vi "Untitled 1.vi"() -> ()   [LabVIEW 2020]
uses:
  <vilib>/Instr/_visa.llb/VISA Configure Serial Port (Instr).vi
panel:
  out "z":string
  out "y":string
  out "x":string
  out "y":i32(graph)
  out "x":i32(graph)
  out "z":i32=61
  out "y":i32=61
  out "z":i32(graph)
  in  "等待时间(ms)":u32=200
  out "缓存区":string="23161"
  in  "字节数(5)":u32=5
  in  "开关":bool=TRUE
  out "x":i32=61
  out "错误输出":cluster{"status":bool, i32, string}={"status"=FALSE, 1073676294, "VISA Read in Untitled 1.vi"}
  in  "串口":refnum<visa-resource-name>="COM4"
  in  "串口设置":T1={"流控制 (0:none)"=0, "停止位 (10: 1 bit)"=10, "奇偶校验 (0:none)"=0, "数据比特 (8)"=8, "比特率 (115200)"=115200} {"数据比特 (8)" min=5 max=8 step=1; "奇偶校验 (0:none)" items=["None", "Odd", "Even", "Mark", "Space"]; "流控制 (0:none)" items=["None", "XON/XOFF", "RTS/CTS", "XON/XOFF & RTS/CTS", "DTR/DSR", "XON/XOFF & DTR/DSR"]}
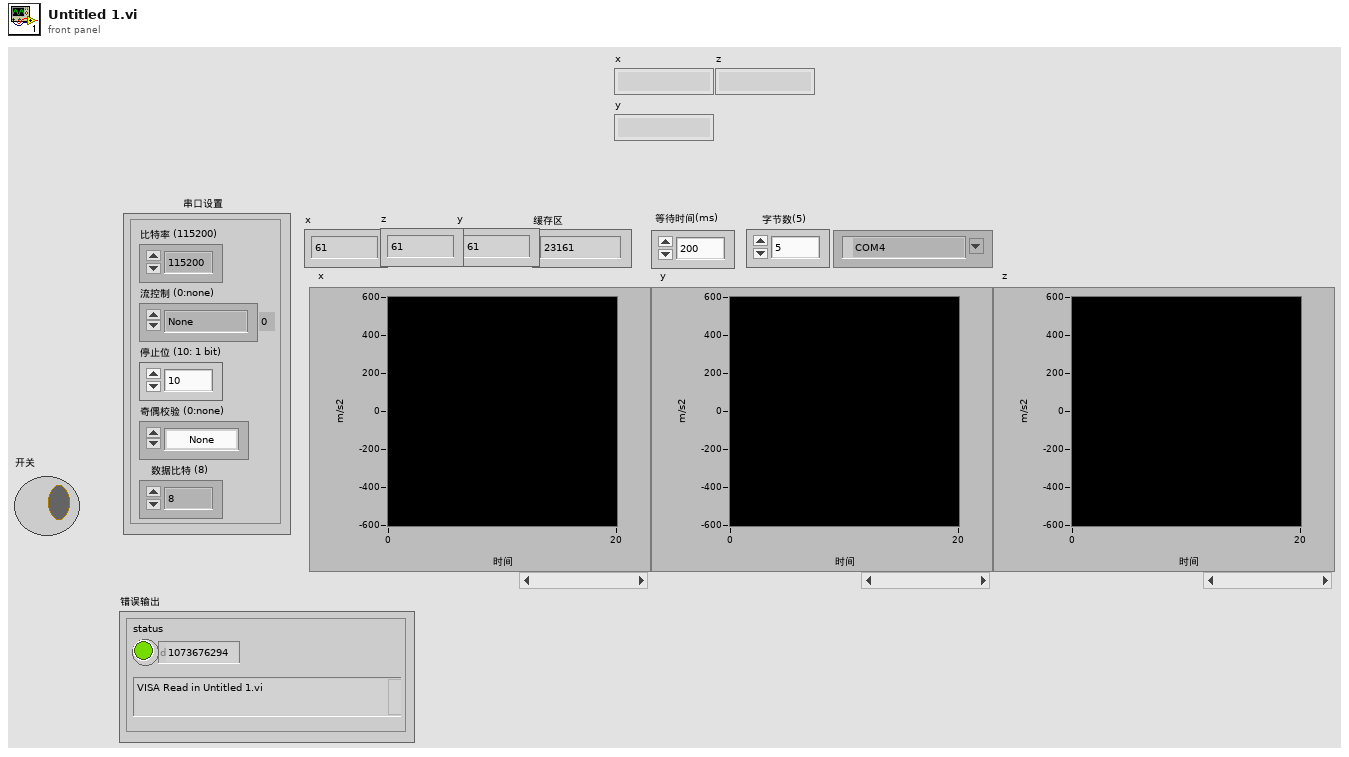
[diagram p1: front panel]
types:
  T1 = cluster{"流控制 (0:none)":u16, "停止位 (10: 1 bit)":u16, "奇偶校验 (0:none)":u16, "数据比特 (8)":u16, "比特率 (115200)":u32}
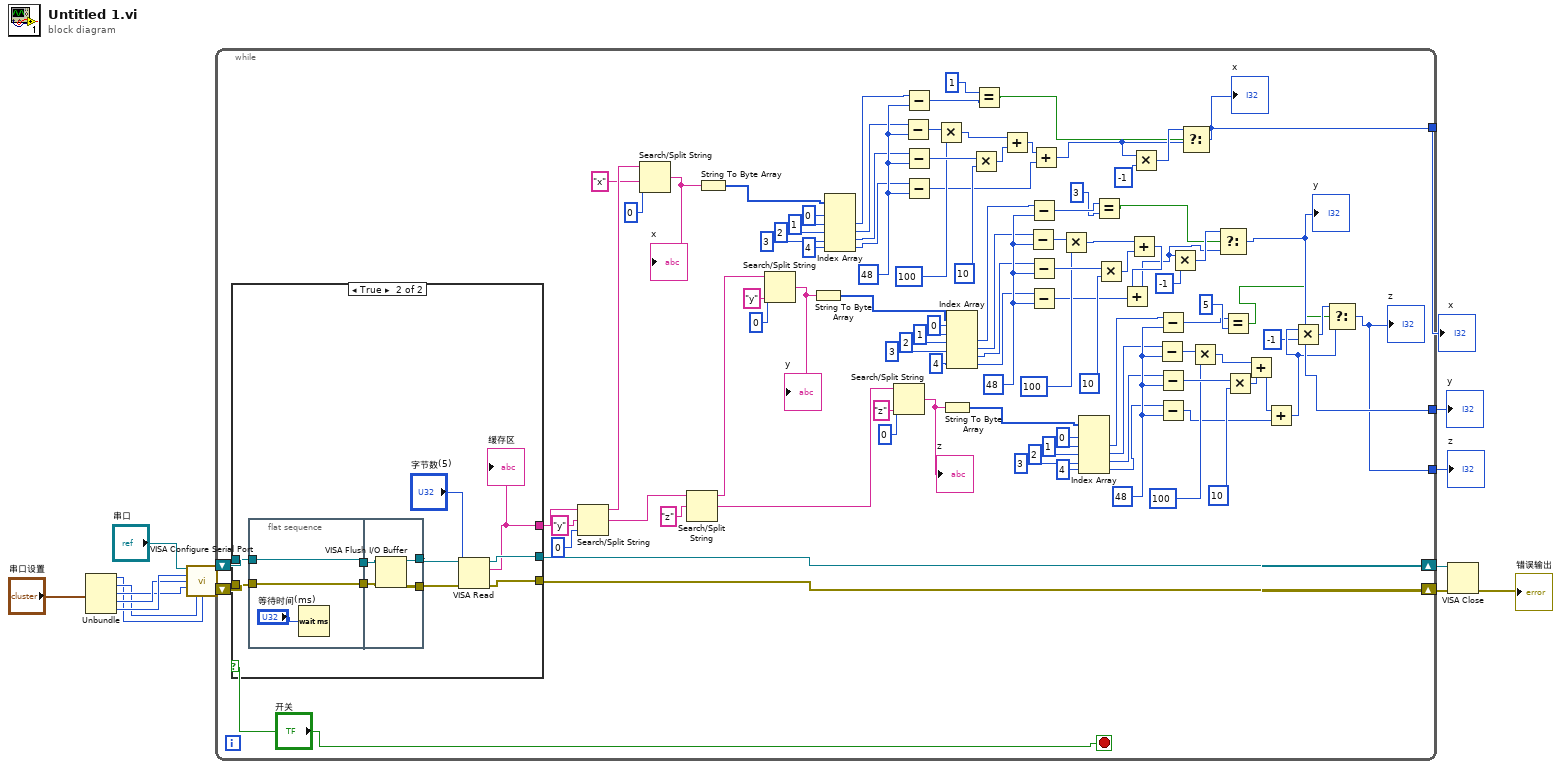
[diagram p0: block diagram]
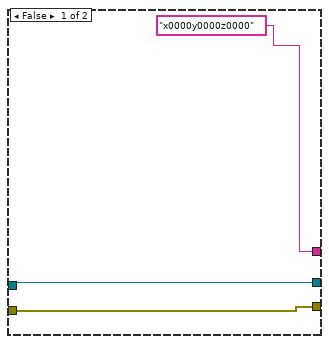
[diagram p2: hidden frame]
diagram:
  n1 = Unbundle("串口设置") -> ("流控制 (0:none)"=w7:u16, "停止位 (10: 1 bit)"=w8:u16, "奇偶校验 (0:none)"=w9:u16, "数据比特 (8)"=w10:u16, "比特率 (115200)"=w11:u32)
  n2 = call-poly "VISA Configure Serial Port"("VISA resource name"="串口", "baud rate (9600)"=w11, "data bits (8)"=w10, "parity (0:none)"=w9, "stop bits (10: 1 bit)"=w8, "flow control (0:none)"=w7) -> ("VISA resource name out"=w15:refnum<visa-resource-name>, "error out"=w14:errorcluster)  [unwired: 8 in]
  n3 = while {
    shift-right: [w112] -> w5
    shift-left: w15 -> [w115]
    shift-right: [w113] -> w6
    shift-left: w14 -> [w114]
    tunnel: [w53] -> w3
    tunnel: [w52] -> w2
    tunnel: [w51] -> w1
    stop <- "开关" stop-if-true
    w72 = 48
    w87 = 48
    w105 = 48
    n4 = case shown="True" "开关" {
      tunnel: w115 -> [w118 w126]
      tunnel: w114 -> [w117 w125]
      tunnel: [w117 w124] -> w113
      tunnel: [w118 w123] -> w112
      tunnel: ["x0000y0000z0000" ("read buffer") w119] -> w98
      frame False {
      }
      frame True {
        n5 = flat-sequence {
          tunnel: [w131] -> w128
          tunnel: w126 -> [w131]
          tunnel: w125 -> [w130]
          tunnel: [w130] -> w127
          tunnel: [w135] -> w121
          tunnel: w128 -> [w134]
          tunnel: w127 -> [w133]
          tunnel: [w132] -> w122
          frame #0 {
            n6 = Wait (ms)(milliseconds to wait="等待时间(ms)") -> ()  [unwired: 1 out]
          }
          frame #1 {
            n7 = VISA Flush I/O Buffer(VISA resource name=w134, error in (no error)=w133) -> (VISA resource name out=w135:refnum<visa-resource-name>, error out=w132:errorcluster)  [unwired: 1 in]
          }
        }
        n8 = VISA Read(VISA resource name=w121, byte count="字节数(5)", error in (no error)=w122) -> (VISA resource name out=w123:refnum<visa-resource-name>, read buffer=w119:string, error out=w124:errorcluster)  [unwired: 1 out]
        "缓存区" <- w119
      }
    }
    n9 = Search/Split String(string=w98, search string/char (-)="y", offset (0)=0) -> (substring before match=w95:string, match + rest of string=w62:string)  [unwired: 1 out]
    n10 = Search/Split String(string=w95, search string/char (-)="x", offset (0)=0) -> (match + rest of string=w40:string)  [unwired: 2 out]
    "x" <- w40
    n11 = Search/Split String(string=w62, search string/char (-)="z") -> (substring before match=w60:string, match + rest of string=w59:string)  [unwired: 1 in, 1 out]
    n12 = String To Byte Array(string=w40) -> (unsigned byte array=w106:u8[])
    n13 = Search/Split String(string=w60, search string/char (-)="y", offset (0)=0) -> (match + rest of string=w78:string)  [unwired: 2 out]
    "y" <- w78
    n14 = String To Byte Array(string=w78) -> (unsigned byte array=w88:u8[])
    n15 = Index Array(array=w106, index #1=0 ("index"), index #2=1 ("index"), index #3=2 ("index"), index #4=3 ("index"), index #5=4 ("index")) -> (element #2=w36:u8, element #3=w35:u8, element #4=w33:u8, element #5=w34:u8)  [unwired: 1 out]
    n16 = Search/Split String(string=w59, search string/char (-)="z", offset (0)=0) -> (match + rest of string=w63:string)  [unwired: 2 out]
    "z" <- w63
    n17 = Subtract(x=w35, y=w105) -> (x-y=w104:i32)
    n18 = Subtract(x=w36, y=w105) -> (x-y=w23:i32)
    n19 = Subtract(x=w33, y=w105) -> (x-y=w103:i32)
    n20 = Subtract(x=w34, y=w105) -> (x-y=w50:i32)
    n21 = Multiply(x=w104, y=100) -> (x*y=w100:i32)
    n22 = String To Byte Array(string=w63) -> (unsigned byte array=w73:u8[])
    n23 = Index Array(array=w88, index #1=0 ("index"), index #2=1 ("index"), index #3=2 ("index"), index #4=3 ("index"), index #5=4 ("index")) -> (element #2=w32:u8, element #3=w31:u8, element #4=w30:u8, element #5=w29:u8)  [unwired: 1 out]
    n24 = Multiply(x=w103, y=10) -> (x*y=w99:i32)
    n25 = Equal?(x=1 ("y"), y=w23) -> (x = y?=w22:bool)
    n26 = Add(x=w100, y=w99) -> (x+y=w49:i32)
    n27 = Subtract(x=w31, y=w87) -> (x-y=w86:i32)
    n28 = Subtract(x=w32, y=w87) -> (x-y=w21:i32)
    n29 = Subtract(x=w30, y=w87) -> (x-y=w85:i32)
    n30 = Subtract(x=w29, y=w87) -> (x-y=w47:i32)
    n31 = Add(x=w49, y=w50) -> (x+y=w48:i32)
    n32 = Multiply(x=w86, y=100) -> (x*y=w82:i32)
    n33 = Index Array(array=w73, index #1=0 ("index"), index #2=1 ("index"), index #3=2 ("index"), index #4=3 ("index"), index #5=4 ("index")) -> (element #2=w28:u8, element #3=w27:u8, element #4=w26:u8, element #5=w25:u8)  [unwired: 1 out]
    n34 = Equal?(x=w21, y=3) -> (x = y?=w19:bool)
    n35 = Multiply(x=w85, y=10) -> (x*y=w81:i32)
    n36 = Add(x=w82, y=w81) -> (x+y=w46:i32)
    n37 = Add(x=w46, y=w47) -> (x+y=w45:i32)
    n38 = Multiply(x=w48, y=-1) -> (x*y=w57:i32)
    n39 = Subtract(x=w27, y=w72) -> (x-y=w71:i32)
    n40 = Subtract(x=w28, y=w72) -> (x-y=w16:i32)
    n41 = Subtract(x=w26, y=w72) -> (x-y=w70:i32)
    n42 = Subtract(x=w25, y=w72) -> (x-y=w44:i32)
    n43 = Multiply(x=w45, y=-1) -> (x*y=w56:i32)
    n44 = Select(t=w57, s=w22, f=w48) -> (s? t:f=w53:i32)
    "x" <- w53
    n45 = Multiply(x=w71, y=100) -> (x*y=w67:i32)
    n46 = Select(t=w56, s=w19, f=w45) -> (s? t:f=w52:i32)
    "y" <- w52
    n47 = Equal?(x=w16, y=5) -> (x = y?=w18:bool)
    n48 = Multiply(x=w70, y=10) -> (x*y=w66:i32)
    n49 = Add(x=w67, y=w66) -> (x+y=w43:i32)
    n50 = Add(x=w43, y=w44) -> (x+y=w42:i32)
    n51 = Multiply(x=w42, y=-1) -> (x*y=w54:i32)
    n52 = Select(t=w54, s=w18, f=w42) -> (s? t:f=w51:i32)
    "z" <- w51
  }
  "z" <- w1
  "x" <- w3
  "y" <- w2
  n53 = VISA Close(VISA resource name=w5, error in (no error)=w6) -> (error out=→"错误输出":errorcluster)
